vi "Do.vi"(8 "error in (no error)":errorcluster, 10 "Actor in":refnum<class "Actor.lvclass">, 11 "send response Msg":refnum<class "send response Msg.lvclass">) -> (0 "error out":errorcluster, 2 "Actor out":refnum<class "Actor.lvclass">)   [LabVIEW 2025, in "send response Msg.lvclass"]
doc: "This VI delivers the message to the actor by calling the appropriate method(s) on the actor."
uses:
  send response Msg.lvclass
  <vilib>/ActorFramework/Actor/Actor.lvclass
  send response Msg.lvclass/send response Msg.ctl
  Send Notification/Send Notification.lvclass
  9ef47adc-f318-494c-9b8b-6df3216d6863.vi
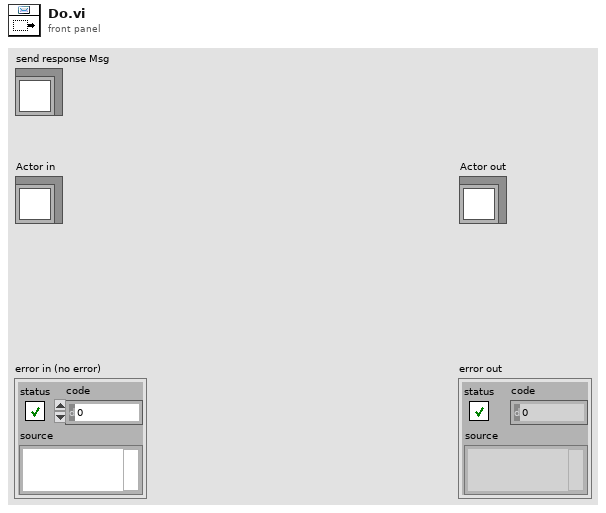
[diagram p1: front panel]
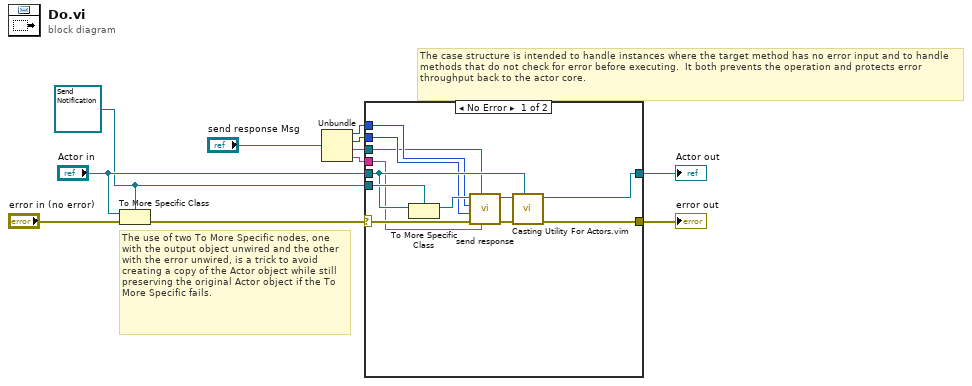
[diagram p0: block diagram]
diagram:
  w5 = refnum<class "Send Notification.lvclass"> refnum ("Actor in")
  # "The use of two To More Specific nodes, one with the output object unwired and the other with the error unwired, is a trick to avoid creating a copy of the Actor object while still preserving the original Actor object if the To More Specific fails."
  # "The case structure is intended to handle instances where the target method has no error input and to handle methods that do not check for error before executing.  It both prevents the operation and protects error throughput back to the actor core."
  n1 = To More Specific Class(target class=w5, reference="Actor in", error in="error in (no error)") -> (error out=w9:errorcluster)  [unwired: 1 out]
  n2 = Unbundle("send response Msg") -> (w4:u32, w3:u16, w2:refnum<k16>, w1:string)
  n3 = case shown="No Error" w9 {
    selector: w9 -> [w23 w25]
    tunnel: [w17 w25] -> w8
    tunnel: [w18 w24] -> w7
    tunnel: "Actor in" -> [w20 w24]
    tunnel: w5 -> [w21 _]
    tunnel: w4 -> [w15 _]
    tunnel: w3 -> [w14 _]
    tunnel: w2 -> [w13 _]
    tunnel: w1 -> [w12 _]
    frame No Error {
      n4 = To More Specific Class(target class=w21, reference=w20) -> (specific class reference=w22:refnum<class "Send Notification.lvclass">)  [unwired: 1 in, 1 out]
      n5 = call-dynamic "send response.vi"("udp message"=w12, "connection ID out"=w13, "error in (no error)"=w23, "port"=w14, "address"=w15, "Send Notification in"=w22) -> ("error out"=w16:errorcluster, "Send Notification out"=w19:refnum<class "Send Notification.lvclass">)  [unwired: 4 in]
      n6 = call "Casting Utility For Actors.vim"("type"=w20, "error in (no error)"=w16, "Actor in"=w19) -> ("error out"=w17:errorcluster, "Actor out"=w18:refnum<class "Actor.lvclass">)  [unwired: 7 in]
    }
    frame Error {
      # "If type check fails, pass the original object out again."
    }
  }
  "error out" <- w8
  "Actor out" <- w7
